vi "XY Graph Init.vi"(4 "Graph Tool Panels Visibility":T1={"Scale Legend Vis"=TRUE, "X-Scrollbar Vis"=FALSE, "Cursor Panel Vis"=FALSE, "Graph Palette Vis"=TRUE}, 6 "Max Legend Size (8)":i32=8, 8 "Error In":errorcluster, 9 "Plots to Skip (none)":i32[](array[numeric]), 10 "Metadata Type":variant, 11 "XYGraph in":T2) -> (0 "Error Out":errorcluster)   [LabVIEW 2019, in "XY Graph Add-Ons.lvlib"]
doc: "Clears Plot Names and restores their visibility"
uses:
  XY Graph Add-Ons.lvlib
  XY Graph Refnum.ctl
  XY Graph Tool Panels Visibility.ctl
  XY Graph Property Tag List.ctl
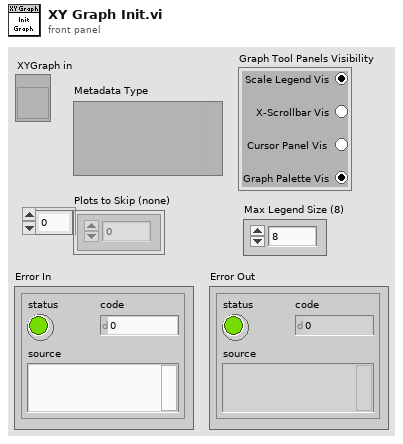
[diagram p1: front panel]
types:
  T1 = typedef "XY Graph Add-Ons.lvlib/XY Graph Tool Panels Visibility.ctl" = cluster{"Scale Legend Vis":bool, "X-Scrollbar Vis":bool, "Cursor Panel Vis":bool, "Graph Palette Vis":bool}
  T2 = typedef "XY Graph Add-Ons.lvlib/XY Graph Refnum.ctl" = refnum<vi>
  T3 = typedef "XY Graph Add-Ons.lvlib/XY Graph Property Tag List.ctl" = enum16{"Max Legend Size", "Preserved Plots", "XScales.GridColors", "YScales.GridColors", "TipStrip String", "TipStrip Visible", "Tool Panels Visibility", "Plots Metadata"}
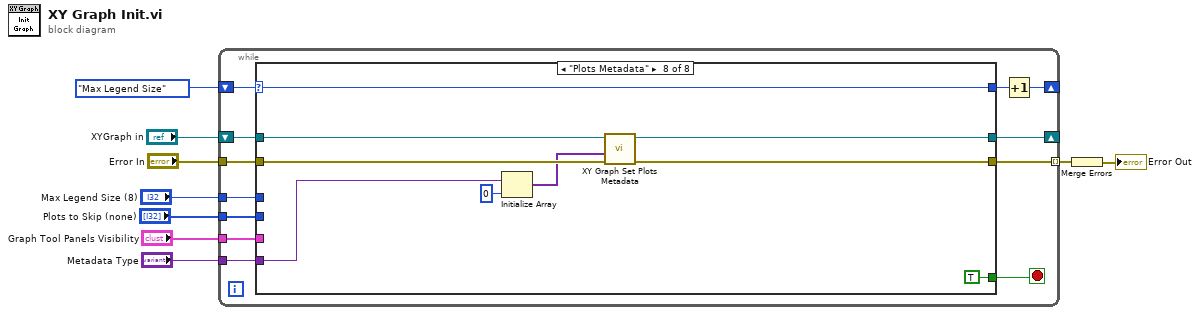
[diagram p0: block diagram]
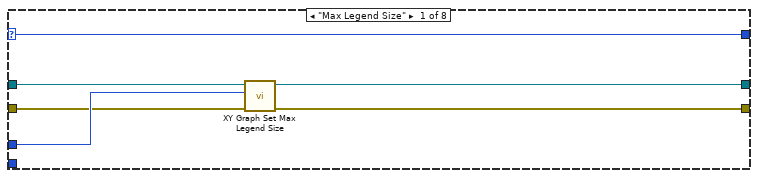
[diagram p2: hidden frame]
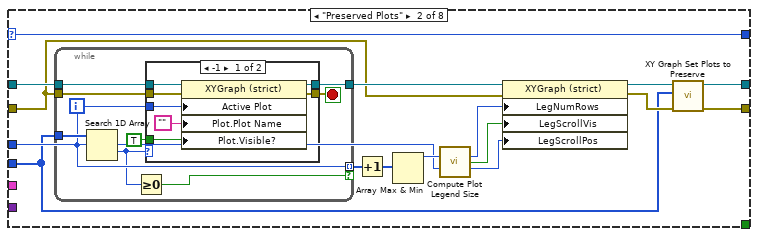
[diagram p3: hidden frame]
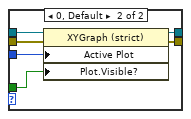
[diagram p4: hidden frame]
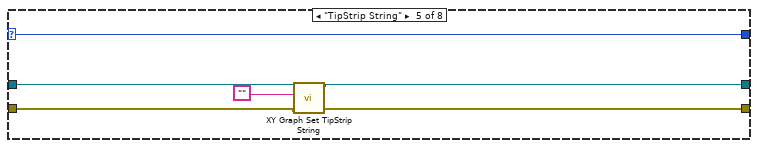
[diagram p7: hidden frame]
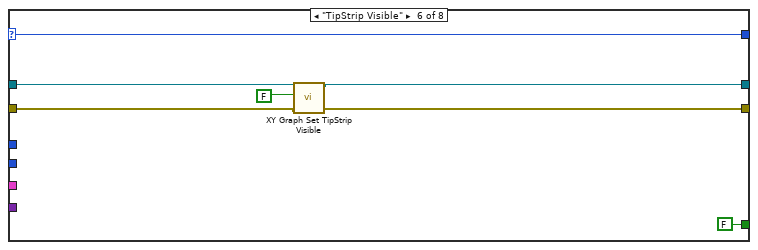
[diagram p8: hidden frame]
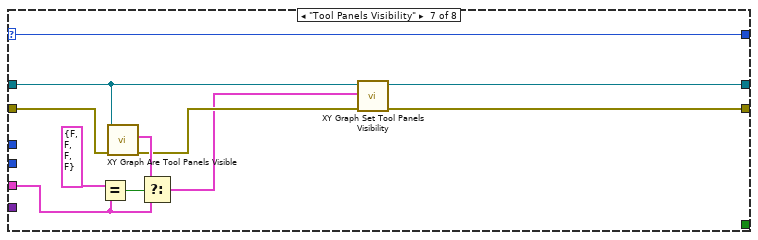
[diagram p9: hidden frame]
diagram:
  n1 = while {
    tunnel: "Error In" -> [w20]
    tunnel: "Plots to Skip (none)" -> [w19]
    tunnel: "Max Legend Size (8)" -> [w18]
    shift-right: [w15] -> _
    shift-left: XY_Graph_Property_Tag_List."Max Legend Size" ("XY Graph Property Tag") -> [w17]
    shift-right: [w13] -> _
    shift-left: "XYGraph in" -> [w21]
    tunnel: [w12] -> w4 mode=indexing
    tunnel: "Graph Tool Panels Visibility" -> [w11]
    tunnel: "Metadata Type" -> [w10]
    stop <- w14 stop-if-true
    n2 = case shown="\"Plots Metadata\"" w17 {
      selector: w17 -> [w27 w33 w67 w70 w77 w84 w95 w104]
      tunnel: w21 -> [w25 w43 w68 w71 w76 w83 w91 w100]
      tunnel: w20 -> [w23 w39 w66 w69 w75 w82 w88 w99]
      tunnel: w19 -> [_ w28 _ _ _ _ _ _]
      tunnel: w18 -> [w26 w34 _ _ _ _ _ _]
      tunnel: [w27 w33 w67 w70 w77 w84 w95 w104] -> w16
      tunnel: [_ _ _ _ _ FALSE _ TRUE] -> w14
      tunnel: [w24 w29 w68 w71 w74 w81 w94 w103] -> w13
      tunnel: [w22 w30 w66 w69 w73 w80 w93 w102] -> w12
      tunnel: w11 -> [_ _ _ _ _ _ w85 _]
      tunnel: w10 -> [_ _ _ _ _ _ _ w98]
      frame "Max Legend Size" {
        n3 = call "XY Graph Set Max Legend Size.vi"("error in (no error)"=w23, "Max Legend Size"=w26, "XY Graph Refnum"=w25) -> ("error out"=w22:errorcluster, "XY Graph Refnum (dup)"=w24:T2)  [unwired: 7 in]
      }
      frame "Preserved Plots" {
        n4 = while {
          tunnel: w43 -> [w52]
          tunnel: w39 -> [w50]
          tunnel: w28 -> [w49]
          tunnel: [w47] -> w42 mode=indexing if=w45
          tunnel: [w44] -> w40
          i -> [w47]
          stop <- w51 stop-if-true
          n5 = Search 1D Array(1D array=w49, element=w47) -> (index of element=w46:i32)  [unwired: 1 in]
          n6 = Greater Or Equal To 0?(x=w46) -> (x >= 0?=w45:bool)
          n7 = case shown="-1" w46 {
            tunnel: w52 -> [w59 w63]
            tunnel: [w58 w62] -> w51
            tunnel: w50 -> [w57 w64]
            tunnel: w47 -> [w56 w65]
            tunnel: TRUE ("Plot.Visible") -> [w54 w61]
            tunnel: [w53 w60] -> w44
            frame -1 {
              n8 = property class="XYGraph (strict)"(reference=w59, error in=w57, "Active Plot"=w56, "Plot.Plot Name"="", "Plot.Visible?"=w54) -> (reference out=w53:T2, error out=w58:errorcluster)
            }
            frame 0, Default {
              n9 = property class="XYGraph (strict)"(reference=w63, error in=w64, "Active Plot"=w65, "Plot.Visible?"=w61) -> (reference out=w60:T2, error out=w62:errorcluster)
            }
          }
        }
        n10 = Increment(x=w42) -> (x+1=w41:i32[])
        n11 = Array Max & Min(array=w41) -> (max value=w38:i32)  [unwired: 3 out]
        n12 = call "Compute Plot Legend Size.vi"("# Plots"=w38, "Max Legend Size"=w34) -> ("LegNumRows"=w37:u32, "LegScrollVis"=w36:bool, "LegScrollPos"=w35:u32)  [unwired: 11 in]
        n13 = property class="XYGraph (strict)"(reference=w40, error in=w39, "LegNumRows"=w37, "LegScrollVis"=w36, "LegScrollPos"=w35) -> (reference out=w32:T2, error out=w31:errorcluster)
        n14 = call "XY Graph Set Plots to Preserve.vi"("error in (no error)"=w31, "Plots to Preserve"=w28, "XY Graph Refnum"=w32) -> ("error out"=w30:errorcluster, "XY Graph Refnum (dup)"=w29:T2)  [unwired: 7 in]
      }
      frame "XScales.GridColors" {
      }
      frame "YScales.GridColors" {
      }
      frame "TipStrip String" {
        n15 = call "XY Graph Set TipStrip String.vi"("error in (no error)"=w75, "TipStrip String"="", "XY Graph Refnum"=w76) -> ("error out"=w73:errorcluster, "XY Graph Refnum (dup)"=w74:T2)  [unwired: 6 in, 1 out]
      }
      frame "TipStrip Visible" {
        n16 = call "XY Graph Set TipStrip Visible.vi"("error in (no error)"=w82, "TipStrip Visible"=FALSE, "XY Graph Refnum"=w83) -> ("error out"=w80:errorcluster, "XY Graph Refnum (dup)"=w81:T2)  [unwired: 6 in, 1 out]
      }
      frame "Tool Panels Visibility" {
        n17 = Equal?(x=T1 {"Scale Legend Vis"=FALSE, "X-Scrollbar Vis"=FALSE, "Cursor Panel Vis"=FALSE, "Graph Palette Vis"=FALSE} ("y"), y=w85) -> (x = y?=w92:bool)
        n18 = call "XY Graph Are Tool Panels Visible.vi"("Error In"=w88, "XY Graph Ref"=w91) -> ("Error Out"=w89:errorcluster, "Graph Tool Panels Visibility"=w90:T1)  [unwired: 7 in, 1 out]
        n19 = Select(t=w90, s=w92, f=w85) -> (s? t:f=w87:T1)
        n20 = call "XY Graph Set Tool Panels Visibility.vi"("error in (no error)"=w89, "Graph Tool Panels Visibility"=w87, "XYGraph in"=w91) -> ("error out"=w93:errorcluster, "XYGraph out"=w94:T2)  [unwired: 7 in]
      }
      frame "Plots Metadata" {
        n21 = Initialize Array(w98, 0 ("dimension size")) -> (w96:variant[])
        n22 = call "XY Graph Set Plots Metadata.vi"("error in (no error)"=w99, "Plots Metadata"=w96, "XY Graph Refnum"=w100) -> ("error out"=w102:errorcluster, "XY Graph Refnum (dup)"=w103:T2)  [unwired: 7 in]
      }
    }
    n23 = Increment(x=w16) -> (x+1=w15:T3)
  }
  n24 = Merge Errors(w4) -> (→"Error Out":errorcluster)
